vi "Path to Wheel Path.vi"(10 "Wheelbase (in)":dbl, 11 "waypoints":cluster{"x":dbl[], "y":dbl[]}) -> (3 "out":cluster{dbl[], dbl[]}[](array[cluster]))   [LabVIEW 2019]
uses:
  <vilib>/Analysis/_algsub.llb/Vector Norm Type.ctl
  <vilib>/Analysis/baseanly.llb/Unit Vector (DBL).vi
  <vilib>/Analysis/baseanly.llb/Real A x B.vi
  <vilib>/Analysis/NI_AALBase.lvlib
  <vilib>/Analysis/NI_AALPro.lvlib
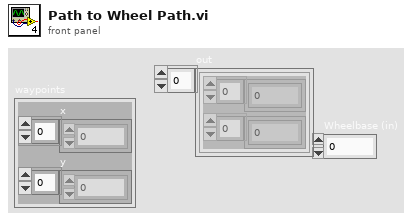
[diagram p1: front panel]
types:
  T1 = typedef "NI_AALPro.lvlib/Vector Norm Type.ctl" = u16
  T2 = typedef "NI_Matrix.lvlib/RealMatrix.ctl" = dbl[][]
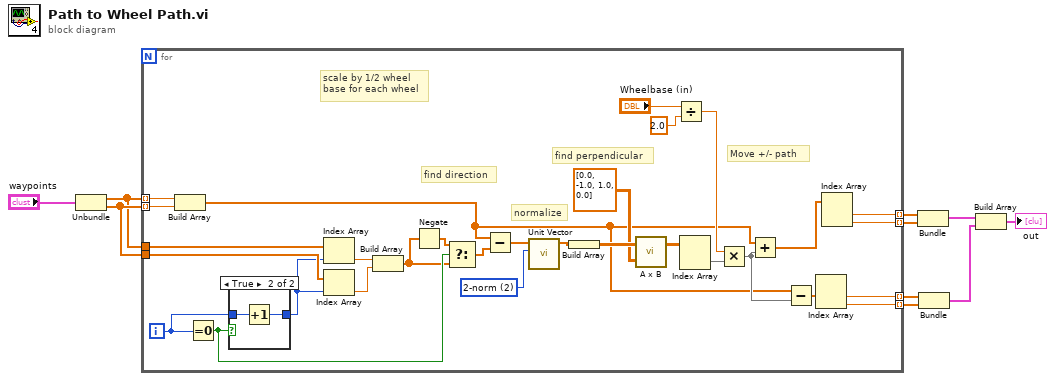
[diagram p0: block diagram]
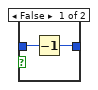
[diagram p2: hidden frame]
diagram:
  n1 = Unbundle("waypoints") -> ("x"=w9:dbl[], "y"=w10:dbl[])
  n2 = for {
    tunnel: w9 -> [w27] mode=indexing
    tunnel: w10 -> [w28] mode=indexing
    tunnel: w10 -> [w39]
    tunnel: w9 -> [w40]
    tunnel: [w32] -> w8 mode=indexing
    tunnel: [w31] -> w7 mode=indexing
    tunnel: [w30] -> w5 mode=indexing
    tunnel: [w29] -> w6 mode=indexing
    i -> [w14]
    w11 = T1 2 items=["1-norm"=1, "2-norm"=2, "Inf-norm"=3, "-Inf-norm"=4, "User Defined"=5] ("norm type")
    # "Move +/- path"
    # "scale by 1/2 wheel\nbase for each wheel"
    # "find perpendicular"
    # "normalize"
    # "find direction"
    n3 = Build Array(w27, w28) -> (w12:dbl[])
    n4 = Equal To 0?(x=w14) -> (x = 0?=w18:bool)
    n5 = case shown="True" w18 {
      tunnel: w14 -> [w41 w44]
      tunnel: [w42 w43] -> w38
      frame False {
        n6 = Decrement(x=w41) -> (x-1=w42:i32)
      }
      frame True {
        n7 = Increment(x=w44) -> (x+1=w43:i32)
      }
    }
    n8 = Index Array(array=w40, index=w38) -> (element=w37:dbl)
    n9 = Index Array(array=w39, index=w38) -> (element=w36:dbl)
    n10 = Build Array(w37, w36) -> (w17:dbl[])
    n11 = Negate(x=w17) -> (-x=w16:dbl[])
    n12 = Select(t=w16, s=w18, f=w17) -> (s? t:f=w19:dbl[])
    n13 = Subtract(x=w12, y=w19) -> (x-y=w23:dbl[])
    n14 = call-poly <vilib>:"Unit Vector.vi"("norm type"=w11, "Input Vector"=w23) -> ("Unit Vector"=w22:dbl[])  [unwired: 7 in, 2 out]
    n15 = Build Array(w22) -> (w26:dbl[][])
    n16 = call-poly <vilib>:"A x B.vi"("B"=dbl[][] [[0.0, -1.0], [1.0, 0.0]], "A"=w26) -> ("A x B"=w20:T2)  [unwired: 1 out]
    n17 = Divide(x="Wheelbase (in)", y=2.0) -> (x/y=w34:dbl)
    n18 = Index Array(array=w20) -> (element=w24:dbl[])  [unwired: 2 in]
    n19 = Multiply(x=w34, y=w24) -> (x*y=w15:dbl[])
    n20 = Add(x=w12, y=w15) -> (x+y=w13:dbl[])
    n21 = Subtract(x=w12, y=w15) -> (x-y=w21:dbl[])
    n22 = Index Array(array=w21) -> (element #1=w29:dbl, element #2=w30:dbl)  [unwired: 2 in]
    n23 = Index Array(array=w13) -> (element #1=w32:dbl, element #2=w31:dbl)  [unwired: 2 in]
  }
  n24 = Bundle(w8, w7) -> (w4:cluster{dbl[], dbl[]})  [unwired: 1 in]
  n25 = Bundle(w6, w5) -> (w3:cluster{dbl[], dbl[]})  [unwired: 1 in]
  n26 = Build Array(w4, w3) -> (→"out":cluster{dbl[], dbl[]}[])
